vi "Save File Look For Header.vi"(8 "Error In":errorcluster, 10 "Summary Header":string[](array[string]), 11 "Full Data IN":string[][](array[string])) -> (0 "Error Out":errorcluster, 3 "Data Out":string[][](array[string]))   [LabVIEW 2016]
panel:
  out "Header Found!":bool
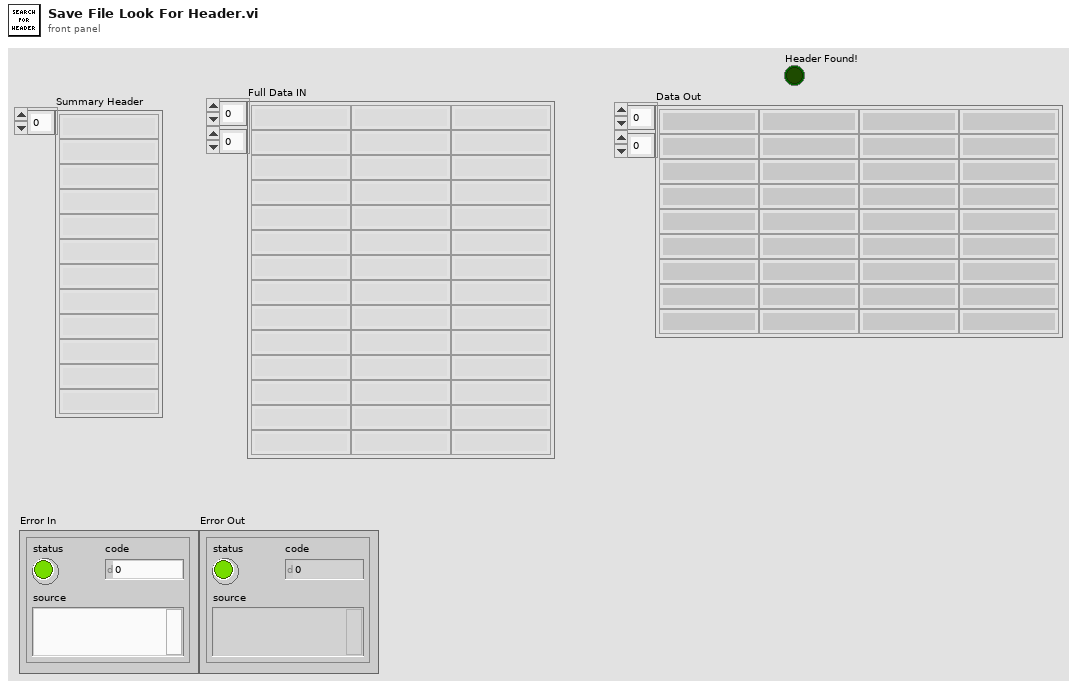
[diagram p1: front panel]
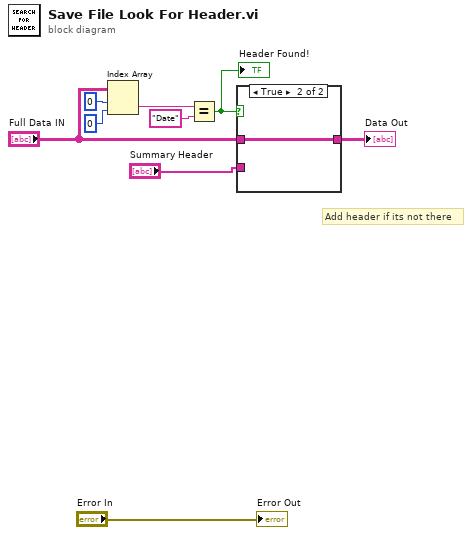
[diagram p0: block diagram]
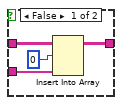
[diagram p2: hidden frame]
diagram:
  # "Add header if its not there"
  n1 = Index Array(array="Full Data IN", index (row)=0, index (col)=0 ("disabled index (col)")) -> (element=w4:string)
  n2 = Equal?(x=w4, y="Date") -> (x = y?=w6:bool)
  "Header Found!" <- w6
  n3 = case shown="True" w6 {
    tunnel: "Full Data IN" -> [w13 w14]
    tunnel: [w11 w14] -> w8
    tunnel: "Summary Header" -> [w10 _]
    frame False {
      n4 = Insert Into Array(array=w13, index (row)=0, new element=w10) -> (w11:string[][])  [unwired: 1 in]
    }
    frame True {
    }
  }
  "Data Out" <- w8
  "Error Out" <- "Error In"
